vi "Reflesh Palette Menu.vi"(8 "error in (no error)":errorcluster, 9 "Run Mode?":bool, 11 "MenuRef":refnum<k9>) -> (0 "error out":errorcluster)   [LabVIEW 2020, in "2D Plot.lvclass"]
uses:
  <vilib>/Math Plots/2D Math Plots/2D Plot/2D Plot/2D Plot.lvclass
panel:
  in  "Edit-time Menu":T1(array[cluster])=[{"menu tag"="", "items to delete"=["APP_SC_VISIBLE_ITEMS", "APP_SEPARATOR", "APP_SC_FIT_CONTROL_TO_PANE", "APP_SC_GROWABLE_OBJECT", "APP_SC_SHOW_LAST_ELEMENT", "APP_SC_SHOW_SELECTION", "APP_SC_START_SELECTION", "APP_SC_END_SELECTION", "APP_SC_SELECT_ALL", "APP_SC_SHOW_ARRAY_ELEMENT", "APP_SC_PROPERTIES", "APP_SC_DESCRIPTION_AND_TIP", "APP_SC_CREATE", "APP_SC_REPLACE", "APP_SC_DATA_OPERATIONS", "APP_SC_ADVANCED"], "new menu"=[{"item names"="Properties", "item tags"="USER_SC_PROPERTIES", "after item"="APP_SC_SEPARATOR"}], "root?"=TRUE}]
  in  "Run-time Menu":T1(array[cluster])=[{"menu tag"="", "items to delete"=["APP_SC_SHOW_DIAGRAM", "APP_SC_INSERT_ELEMENT_BEFORE", "APP_SC_DELETE_ELEMENT"], "new menu"=[], "root?"=TRUE}]
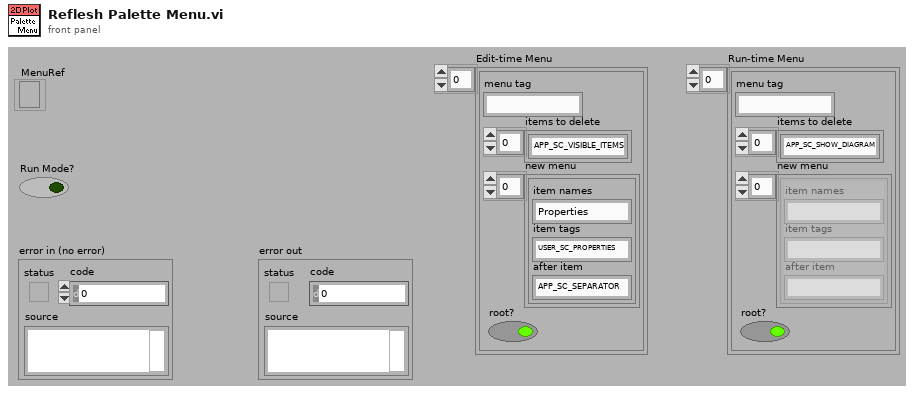
[diagram p1: front panel]
types:
  T1 = cluster{"menu tag":string, "items to delete":string[], "new menu":cluster{"item names":string, "item tags":string, "after item":string}[], "root?":bool}[]
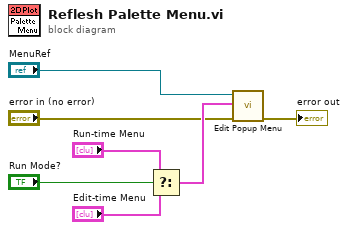
[diagram p0: block diagram]
diagram:
  n1 = Select(t="Run-time Menu", s="Run Mode?", f="Edit-time Menu") -> (s? t:f=w4:T1)
  n2 = call <vilib>:"Edit Popup Menu.vi"("error in (no error)"="error in (no error)", "Menu Operation Cluster"=w4, "Menu Ref In"="MenuRef") -> ("error out"=→"error out":errorcluster)  [unwired: 2 in, 6 out]
